vi "linear ramp new.vi"(0 "Input":T1 {"end value" format="%_6g"; "start value" format="%_6g"; "Ramp end" format="%_6g"; "Ramp begin" format="%_6g"; "DAC Channel" items=["0", "1", "2", "3", "4", "5", "6", "7", "8", "9", "10", "11", "12", "13", "14", "0"]}) -> (1 "Time Array":dbl[](array[numeric]), 2 "Volt Array":dbl[](array[numeric]))   [LabVIEW 2015]
doc: "This VI creates linear DAC ramps and is called from the modules"
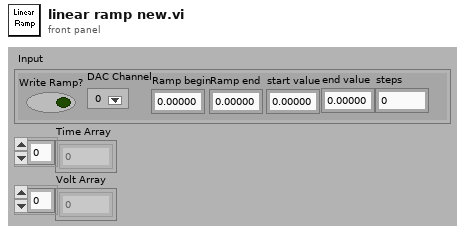
[diagram p1: front panel]
types:
  T1 = cluster{"Write Ramp?":bool, "DAC Channel":i16, "Ramp begin":dbl, "Ramp end":dbl, "start value":dbl, "end value":dbl, "steps":i16}
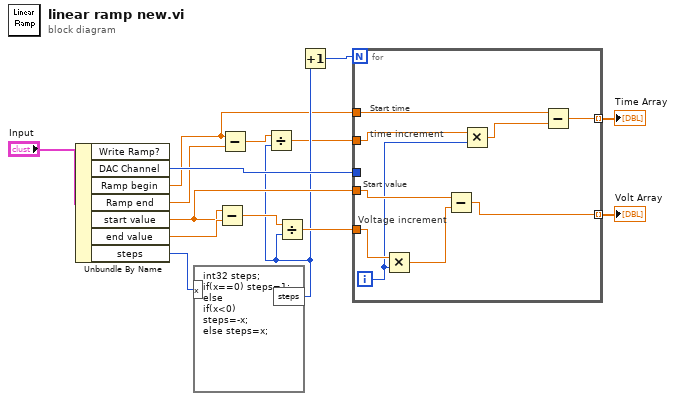
[diagram p0: block diagram]
diagram:
  n1 = Unbundle By Name("Input") -> ("DAC Channel"=w8:i16, "Ramp begin"=w3:dbl, "Ramp end"=w7:dbl, "start value"=w9:dbl, "end value"=w12:dbl, "steps"=w14:i16)  [unwired: 1 out]
  n2 = formula code="int32 steps;\nif(x==0) steps=1;\nelse\nif(x<0)\nsteps=-x;\nelse steps=x;"("x"=w14) -> ("steps"=w5:i32)
  n3 = Subtract(x=w9, y=w12) -> (x-y=w11:dbl)
  n4 = Subtract(x=w3, y=w7) -> (x-y=w6:dbl)
  n5 = Divide(x=w6, y=w5) -> (x/y=w4:dbl)
  n6 = Divide(x=w11, y=w5) -> (x/y=w10:dbl)
  n7 = Increment(x=w5) -> (x+1=w13:i32)
  n8 = for {
    N: w13 -> [_]
    tunnel: w10 -> [w24]
    tunnel: w9 -> [w23]
    tunnel: w8 -> [_]
    tunnel: w4 -> [w21]
    tunnel: w3 -> [w19]
    tunnel: [w17] -> w2 mode=indexing
    tunnel: [w16] -> w1 mode=indexing
    i -> [w20]
    # "time increment"
    # "Start time"
    # "Start value"
    # "Voltage increment"
    n9 = Multiply(x=w24, y=w20) -> (x*y=w22:dbl)
    n10 = Subtract(x=w23, y=w22) -> (x-y=w16:dbl)
    n11 = Multiply(x=w21, y=w20) -> (x*y=w18:dbl)
    n12 = Subtract(x=w19, y=w18) -> (x-y=w17:dbl)
  }
  "Time Array" <- w2
  "Volt Array" <- w1
